vi "I2C Read.vi"(5 "Timeout (1000 ms)":u16=1000, 7 "I2C Channel (0)":u8, 8 "Error In":errorcluster, 9 "Bytes To Read":u8, 10 "I2C Slave Address":u8, 11 "LINX Device Config":T1) -> (0 "Error Out":errorcluster, 2 "Data":u8[](array[numeric]), 3 "LINX Device Config":T1)   [LabVIEW 2013, in "LVH-LINX.lvlib" / "Device.lvlib"]
uses:
  <vilib>/LabVIEW Hacker/LINX/Private/Device/Device.lvlib
  <vilib>/LabVIEW Hacker/LINX/Private/Device/Type Defs/LINX Device Config.ctl
  <vilib>/LabVIEW Hacker/LINX/Private/Type Defs/Interface.ctl
  <vilib>/LabVIEW Hacker/LINX/Private/Device/Type Defs/TCP Config.ctl
  <vilib>/LabVIEW Hacker/LINX/Private/Type Defs/Device Family.ctl
  <vilib>/LabVIEW Hacker/LINX/Private/Type Defs/Error Type.ctl
  <vilib>/LabVIEW Hacker/LINX/LVH-LINX.lvlib
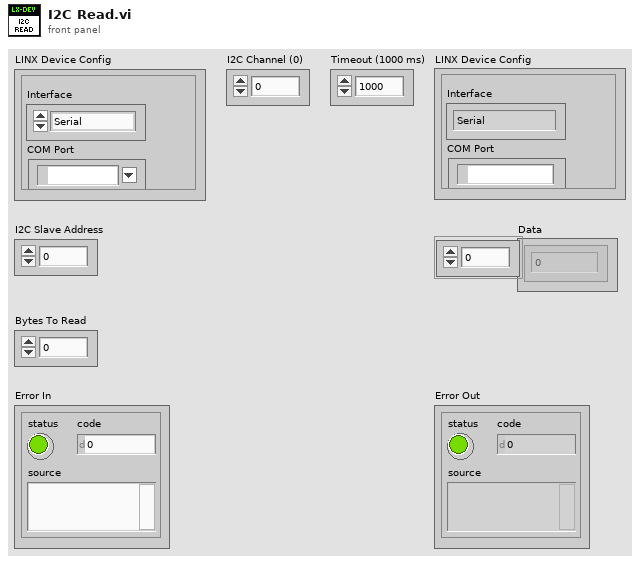
[diagram p1: front panel]
types:
  T1 = typedef "LVH-LINX.lvlib/Device.lvlib/LINX Device Config.ctl" = cluster{"Interface":T2, "COM Port":refnum<visa-resource-name>, "TCP Configuration":T3, "Device Family":T4, "Device ID":u8, "Device Name":string, "TCP Ref":refnum<k5>}
  T2 = typedef "LVH-LINX.lvlib/Interface.ctl" = enum16{"Serial", "TCP"}
  T3 = typedef "LVH-LINX.lvlib/Device.lvlib/TCP Config.ctl" = cluster{"IP Address":string, "Port":u16}
  T4 = typedef "LVH-LINX.lvlib/Device Family.ctl" = enum8{"National Instruments", "Digilent", "Arduino"}
  T5 = typedef "LVH-LINX.lvlib/Error Type.ctl" = enum16{"Unknown", "Timeout", "Corrupt Return Packet", "Unable To Connect", "Command Not Supported", "Channel DNE", "Invalid COM Config"}
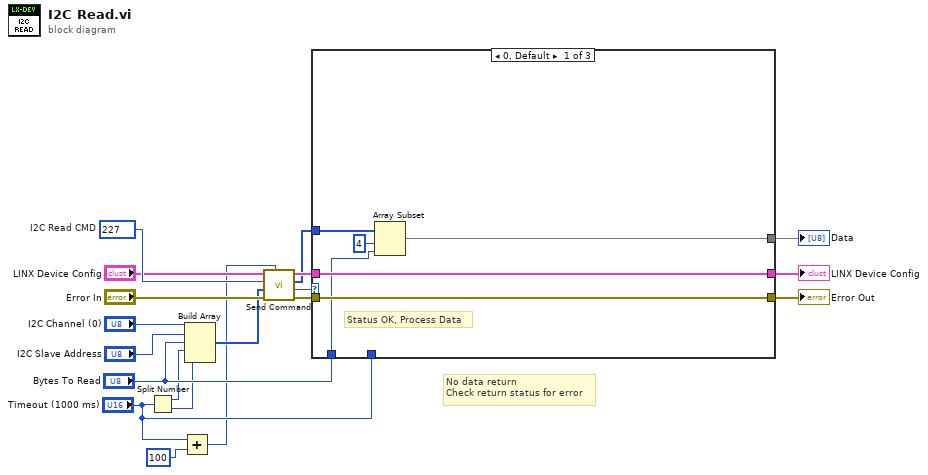
[diagram p0: block diagram]
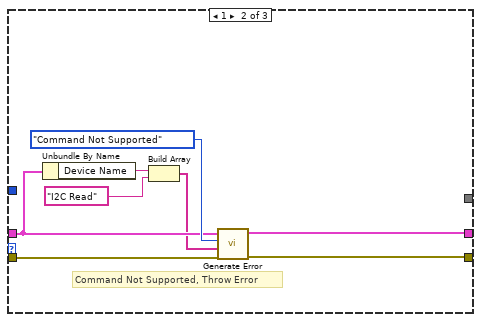
[diagram p2: hidden frame]
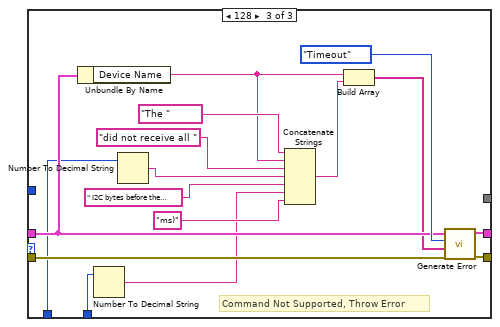
[diagram p3: hidden frame]
diagram:
  w18 = u16 227  # I2C Read CMD
  # "No data return\nCheck return status for error"
  n1 = Split Number(x="Timeout (1000 ms)") -> (hi(x)=w6:u8, lo(x)=w5:u8)
  n2 = Add(x="Timeout (1000 ms)", y=u16 100) -> (x+y=w1:u16)
  n3 = Build Array("I2C Channel (0)", "I2C Slave Address", "Bytes To Read", w6, w5) -> (w11:u8[])
  n4 = call <vilib>:"Send Command.vi"("Timeout (100 ms)"=w1, "Error In"="Error In", "ARGS"=w11, "CMD"=w18, "LINX Device Config"="LINX Device Config") -> ("Error Out"=w13:errorcluster, "Status"=w8:u8, "Response"=w12:u8[], "LINX Device Config"=w15:T1)  [unwired: 3 in]
  n5 = case shown="0, Default" w8 {
    tunnel: [w25 w31 w47] -> w16
    tunnel: w15 -> [w25 w29 w45]
    tunnel: [w24 w32 w48] -> w14
    tunnel: w13 -> [w24 w33 w49]
    tunnel: w12 -> [w23 _ _]
    tunnel: "Bytes To Read" -> [w21 _ w38]
    tunnel: "Timeout (1000 ms)" -> [_ _ w35]
    tunnel: [w20 _ _] -> w4
    frame 0, Default {
      # "Status OK, Process Data"
      n6 = Array Subset(array=w23, index=4, length=w21) -> (w20:u8[])
    }
    frame 1 {
      # "Command Not Supported, Throw Error"
      n7 = Unbundle By Name(w29) -> ("Device Name"=w28:string)
      n8 = Build Array(w28, "I2C Read") -> (w26:string[])
      n9 = call <vilib>:"Generate Error.vi"("Error In"=w33, "Arguments"=w26, "Error Type"=Error_Type."Command Not Supported", "LINX Device Config"=w29) -> ("Error Out"=w32:errorcluster, "LINX Device Config"=w31:T1)  [unwired: 6 in]
    }
    frame 128 {
      # "Command Not Supported, Throw Error"
      n10 = Unbundle By Name(w45) -> ("Device Name"=w39:string)
      n11 = Number To Decimal String(number=w35) -> (decimal integer string=w34:string)  [unwired: 1 in]
      n12 = Number To Decimal String(number=w38) -> (decimal integer string=w36:string)  [unwired: 1 in]
      n13 = Concatenate Strings("The ", w39, "did not receive all " ("string"), w36, " I2C bytes before the specified tiemout (" ("string"), w34, "ms)" ("string")) -> (w40:string)
      n14 = Build Array(w39, w40) -> (w44:string[])
      n15 = call <vilib>:"Generate Error.vi"("Error In"=w49, "Arguments"=w44, "Error Type"=Error_Type."Timeout", "LINX Device Config"=w45) -> ("Error Out"=w48:errorcluster, "LINX Device Config"=w47:T1)  [unwired: 6 in]
    }
  }
  "Error Out" <- w14
  "LINX Device Config" <- w16
  "Data" <- w4
